vi "ConvertTimeConstantString.vi"(8 "error in (no error)":errorcluster, 10 "Time Constant":string) -> (0 "error out":errorcluster, 2 "Time Constant (s)":dbl)   [LabVIEW 2016, in "SR7270 Drivers.lvclass"]
uses:
  SR7270 Drivers.lvclass
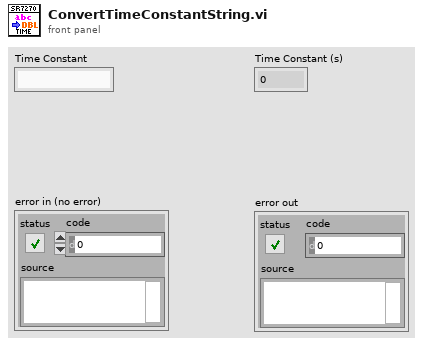
[diagram p1: front panel]
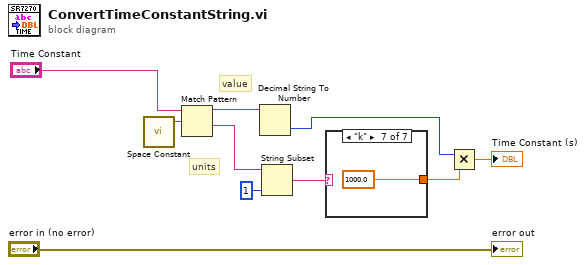
[diagram p0: block diagram]
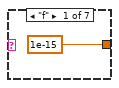
[diagram p2: hidden frame]
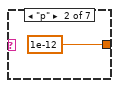
[diagram p3: hidden frame]
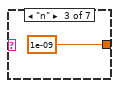
[diagram p4: hidden frame]
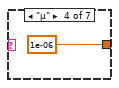
[diagram p5: hidden frame]
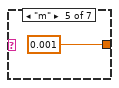
[diagram p6: hidden frame]
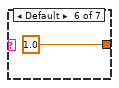
[diagram p7: hidden frame]
diagram:
  # "value"
  # "units"
  n1 = call <vilib>:"Space Constant.vi"() -> ("String"=w10:string)
  n2 = Match Pattern(string="Time Constant", regular expression=w10) -> (before substring=w9:string, after substring=w8:string)  [unwired: 1 in, 2 out]
  n3 = Decimal String To Number(string=w9) -> (number=w4:i32)  [unwired: 2 in, 1 out]
  n4 = String Subset(string=w8, length (rest)=1 ("length (rest)")) -> (substring=w6:string)  [unwired: 1 in]
  n5 = case shown="\"k\"" w6 {
    tunnel: [1e-15 1e-12 1e-09 1e-06 0.001 1.0 1000.0] -> w5
    frame "f" {
    }
    frame "p" {
    }
    frame "n" {
    }
    frame "µ" {
    }
    frame "m" {
    }
    frame Default {
    }
    frame "k" {
    }
  }
  n6 = Multiply(x=w4, y=w5) -> (x*y=→"Time Constant (s)":dbl)
  "error out" <- "error in (no error)"
